vi "Send email notice.vi"(8 "error in (no error)":errorcluster, 10 "Notice type":T1=enum."Tomography error", 11 "Tomo in":refnum<class "Tomo.lvclass">) -> (0 "error out":errorcluster, 3 "Tomo out":refnum<class "Tomo.lvclass">)   [LabVIEW 2012, in "Tomo.lvclass"]
uses:
  Tomo.lvclass
  notice type.ctl
  Tomo.lvclass/Tomo.ctl
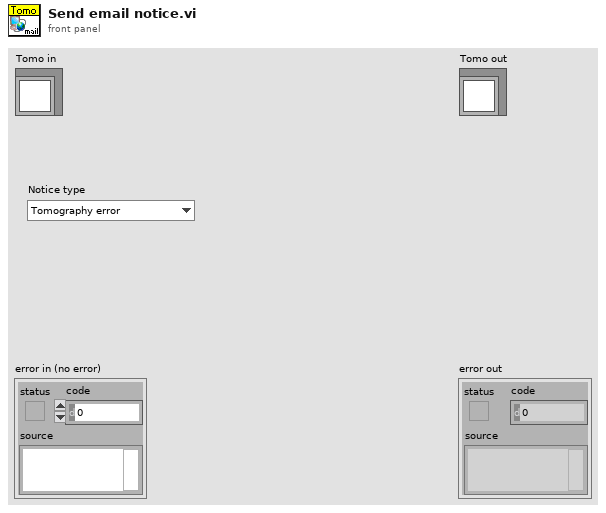
[diagram p1: front panel]
types:
  T1 = typedef "Tomo.lvclass/notice type.ctl" = enum16{"Tomography stopped", "Tomography error", "Tomography finished"}
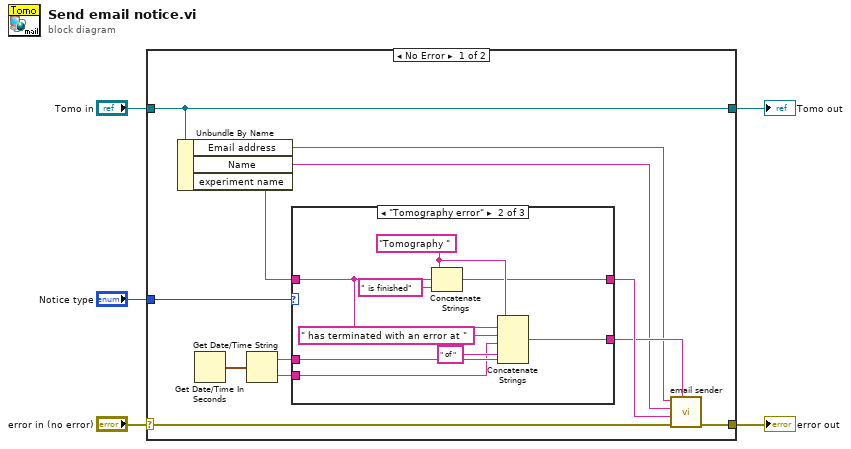
[diagram p0: block diagram]
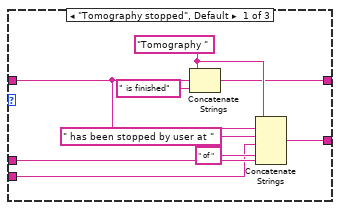
[diagram p2: hidden frame]
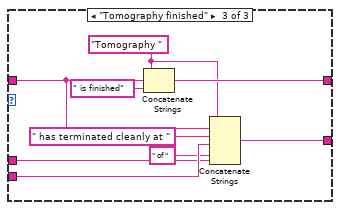
[diagram p3: hidden frame]
diagram:
  n1 = case shown="No Error" "error in (no error)" {
    selector: "error in (no error)" -> [w7 w46]
    tunnel: [w6 w46] -> w4
    tunnel: [w17 w45] -> w2
    tunnel: "Tomo in" -> [w17 w45]
    tunnel: "Notice type" -> [w16 _]
    frame No Error {
      n2 = Unbundle By Name(w17) -> ("Email address"=w9:string, "Name"=w8:string, "experiment name"=w15:string)
      n3 = Get Date/Time In Seconds() -> (seconds since 1Jan1904=w13:timestamp)
      n4 = Get Date/Time String(seconds (now)=w13) -> (date string=w11:string, time string=w12:string)  [unwired: 2 in]
      n5 = case shown="\"Tomography error\"" w16 {
        tunnel: w15 -> [w20 w29 w41]
        tunnel: [w18 w30 w43] -> w14
        tunnel: w12 -> [w21 w27 w39]
        tunnel: w11 -> [w22 w28 w37]
        tunnel: [w19 w31 w36] -> w10
        frame "Tomography stopped", Default {
          w25 = "Tomography " ("string")
          n6 = Concatenate Strings(w25, w20, " is finished" ("string")) -> (w18:string)
          n7 = Concatenate Strings(w25, w20, " has been stopped by user at " ("string"), w21, " of " ("string"), w22) -> (w19:string)
        }
        frame "Tomography error" {
          w33 = "Tomography " ("string")
          n8 = Concatenate Strings(w33, w29, " is finished" ("string")) -> (w30:string)
          n9 = Concatenate Strings(w33, w29, " has terminated with an error at " ("string"), w27, " of " ("string"), w28) -> (w31:string)
        }
        frame "Tomography finished" {
          w42 = "Tomography " ("string")
          n10 = Concatenate Strings(w42, w41, " is finished" ("string")) -> (w43:string)
          n11 = Concatenate Strings(w42, w41, " has terminated cleanly at " ("string"), w39, " of " ("string"), w37) -> (w36:string)
        }
      }
      n12 = call "email sender.vi"("Body"=w10, "error in (no error)"=w7, "Subject"=w14, "Recipient's Name"=w8, "Recipient's Email Address Address"=w9) -> ("error out"=w6:errorcluster)  [unwired: 6 in]
    }
    frame Error {
    }
  }
  "error out" <- w4
  "Tomo out" <- w2
